vi "구획스크롤보이기(subVI).vi"(11 "Pane 입력":refnum<vi>) -> (0 "에러 출력":errorcluster)   [LabVIEW 2014]
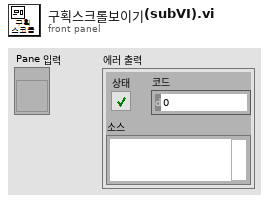
[diagram p1: front panel]
types:
  T1 = enum16{"Always On", "Always Off", "Off While Running"}
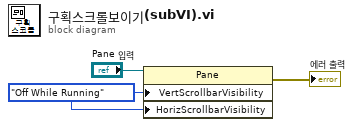
[diagram p0: block diagram]
diagram:
  w2 = T1."Off While Running" ("수직 스크롤 막대 보이기")
  n1 = property on="프로퍼티 노드" class="Pane"(reference="Pane 입력", "VertScrollbarVisibility"=w2, "HorizScrollbarVisibility"=w2) -> (error out=→"에러 출력":errorcluster)  [unwired: 1 in, 1 out]
